vi "RMS (Half Cycle).vi"(0 "waveforms":waveform(dbl)[](array[waveform]), 1 "reset? (F)":bool, 5 "zero crossing":cluster{"zero crossing":dbl[]}[](array[cluster]), 9 "system info in":refnum<class "EP System Info.lvclass">, 11 "error in (no error)":errorcluster) -> (4 "one-cycle RMS":T1(array[cluster]), 6 "half-cycle RMS":T1(array[cluster]), 10 "system info out":refnum<class "EP System Info.lvclass">, 15 "error out":errorcluster)   [LabVIEW 2014, in "NI_EP_Power Quality.lvlib"]
doc: "Calculates the RMS voltage or RMS current for a half/single-cycle block, by using the zero crossings. You can use the Zero Crossing VI to calculate <B>zero crossing</B>. This VI refreshes the RMS values every half-cycle. You use the half/single-cycle RMS values only for detection of voltage dips, swells, and interruption events, detection of rapid voltage changes, and measurement of flickers.\n\nThis VI supports measuring single-line and multiple-line systems."
uses:
  <vilib>/addons/Electrical Power/PQ/NI_EP_Power Quality.lvlib
  <vilib>/addons/Electrical Power/PQ/Common/Classes/System Info/EP System Info.lvclass
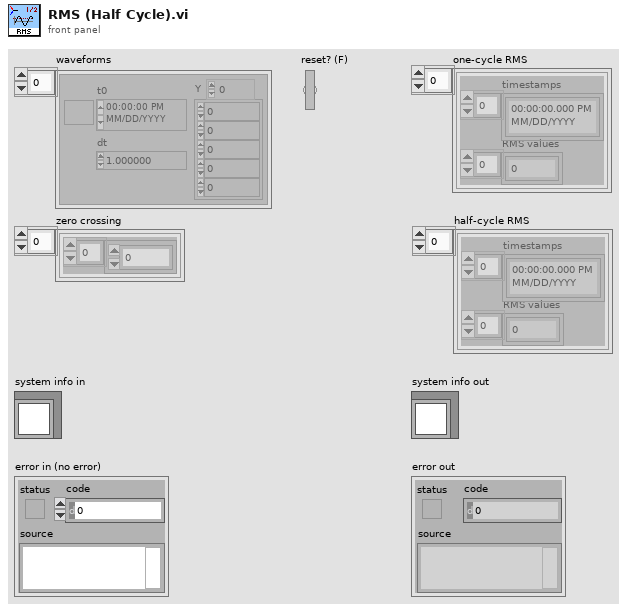
[diagram p1: front panel]
types:
  T1 = cluster{"timestamps":timestamp[], "RMS values":dbl[]}[]
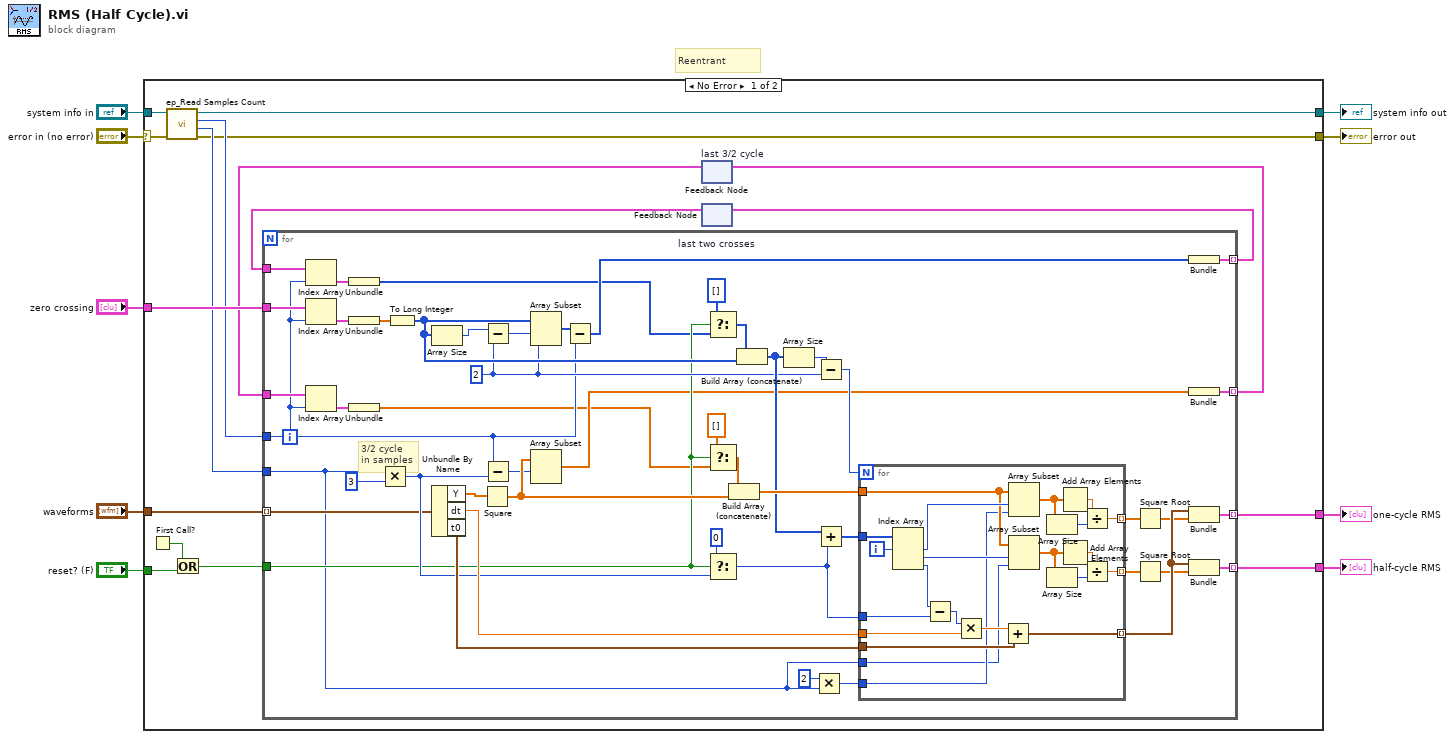
[diagram p0: block diagram]
diagram:
  # "Reentrant"
  n1 = case shown="No Error" "error in (no error)" {
    selector: "error in (no error)" -> [w19 w100]
    tunnel: "waveforms" -> [w26 _]
    tunnel: "system info in" -> [w14 w99]
    tunnel: [w20 w100] -> w5
    tunnel: [w25 _] -> w6
    tunnel: [w24 _] -> w7
    tunnel: "reset? (F)" -> [w11 _]
    tunnel: "zero crossing" -> [w23 _]
    tunnel: [w13 w99] -> w1
    frame No Error {
      n2 = First Call?() -> (First Call?: T/F=w12:bool)
      n3 = call <vilib>:"ep_Read Samples Count.vi"("error in (no error)"=w19, "system info in"=w14) -> ("error out"=w20:errorcluster, "half-cycle (samples)"=w21:i32, "basic calc. interval (samples)"=w22:i32, "system info out"=w13:refnum<class "EP System Info.lvclass">)  [unwired: 5 in, 1 out]
      n4 = Or(x=w12, y=w11) -> (x .or. y?=w10:bool)
      n5 = feedback #1 "last 3/2 cycle"() -> (w15:cluster{dbl[]}[])  [unwired: 1 in]
      n6 = feedback #2 "last two crosses"() -> (w17:cluster{i32[]}[])  [unwired: 1 in]
      n7 = for {
        tunnel: w26 -> [w46] mode=indexing
        tunnel: [w43] -> w24 mode=indexing
        tunnel: [w44] -> w25 mode=indexing
        tunnel: w10 -> [w45]
        tunnel: w23 -> [w49]
        tunnel: w22 -> [w37]
        tunnel: w21 -> [w27]
        tunnel: [w41] -> w18 mode=indexing
        tunnel: w17 -> [w39]
        tunnel: [w35] -> w16 mode=indexing
        tunnel: w15 -> [w33]
        i -> [w32]
        w56 = 2 ("length")
        # "3/2 cycle\nin samples"
        n8 = Index Array(array=w39, index=w32) -> (element=w40:cluster{i32[]})
        n9 = Index Array(array=w49, index=w32) -> (element=w48:cluster{"zero crossing":dbl[]})
        n10 = Index Array(array=w33, index=w32) -> (element=w34:cluster{dbl[]})
        n11 = Unbundle(w40) -> (w38:i32[])
        n12 = Unbundle(w48) -> ("zero crossing"=w47:dbl[])
        n13 = Unbundle(w34) -> (w31:dbl[])
        n14 = Multiply(x=w27, y=3) -> (x*y=w55:i32)
        n15 = To Long Integer(number=w47) -> (32bit integer=w58:i32[])
        n16 = Array Size(array=w58) -> (size(s)=w64:i32)
        n17 = Unbundle By Name(w46) -> ("Y"=w72:dbl[], "dt"=w71:dbl, "t0"=w70:timestamp)
        n18 = Square(x=w72) -> (x^2=w74:dbl[])
        n19 = Subtract(x=w64, y=w56) -> (x-y=w66:i32)
        n20 = Subtract(x=w37, y=w55) -> (x-y=w73:i32)
        n21 = Array Subset(array=w58, index=w66, length=w56) -> (w65:i32[])
        n22 = Array Subset(array=w74, index=w73) -> (w36:dbl[])  [unwired: 1 in]
        n23 = Subtract(x=w65, y=w37) -> (x-y=w42:i32[])
        n24 = Select(t=i32[] [], s=w45, f=w38) -> (s? t:f=w51:i32[])
        n25 = Select(t=dbl[] [], s=w45, f=w31) -> (s? t:f=w53:dbl[])
        n26 = Select(t=0 ("f"), s=w45, f=w55) -> (s? t:f=w59:i32)
        n27 = Build Array (concatenate)(w53, w74) -> (w75:dbl[])
        n28 = Build Array (concatenate)(w51, w58) -> (w61:i32[])
        n29 = Array Size(array=w61) -> (size(s)=w63:i32)
        n30 = Multiply(x=2 ("y"), y=w27) -> (x*y=w28:i32)
        n31 = Subtract(x=w63, y=w56) -> (x-y=w62:i32)
        n32 = Add(x=w61, y=w59) -> (x+y=w60:i32[])
        n33 = for {
          N: w62 -> [_]
          tunnel: w75 -> [w91]
          tunnel: w60 -> [w98]
          tunnel: [w79] -> w69 mode=indexing
          tunnel: [w80] -> w67 mode=indexing
          tunnel: w71 -> [w87]
          tunnel: w70 -> [w85]
          tunnel: [w84] -> w68 mode=indexing
          tunnel: w59 -> [w82]
          tunnel: w28 -> [w78]
          tunnel: w27 -> [w77]
          i -> [w94]
          n34 = Index Array(array=w98, index #1=w94) -> (element #1=w93:i32, element #2=w92:i32, element #3=w83:i32)  [unwired: 2 in]
          n35 = Subtract(x=w83, y=w82) -> (x-y=w81:i32)
          n36 = Multiply(x=w81, y=w87) -> (x*y=w86:dbl)
          n37 = Add(x=w86, y=w85) -> (x+y=w84:timestamp)
          n38 = Array Subset(array=w91, index=w93, length=w78) -> (w97:dbl[])
          n39 = Array Subset(array=w91, index=w92, length=w77) -> (w88:dbl[])
          n40 = Array Size(array=w97) -> (size(s)=w95:i32)
          n41 = Array Size(array=w88) -> (size(s)=w90:i32)
          n42 = Add Array Elements(numeric array=w97) -> (sum=w96:dbl)
          n43 = Add Array Elements(numeric array=w88) -> (sum=w89:dbl)
          n44 = Divide(x=w96, y=w95) -> (x/y=w79:dbl)
          n45 = Divide(x=w89, y=w90) -> (x/y=w80:dbl)
        }
        n46 = Square Root(x=w69) -> (sqrt(x)=w57:dbl[])
        n47 = Square Root(x=w67) -> (sqrt(x)=w30:dbl[])
        n48 = Bundle(w42) -> (w41:cluster{i32[]})  [unwired: 1 in]
        n49 = Bundle(w36) -> (w35:cluster{dbl[]})  [unwired: 1 in]
        n50 = Bundle(w68, w57) -> (w44:cluster{timestamp[], dbl[]})  [unwired: 1 in]
        n51 = Bundle(w68, w30) -> (w43:cluster{timestamp[], dbl[]})  [unwired: 1 in]
      }
      n52 = feedback-in #1(w16) -> ()
      n53 = feedback-in #2(w18) -> ()
    }
    frame Error {
    }
  }
  "error out" <- w5
  "one-cycle RMS" <- w6
  "system info out" <- w1
  "half-cycle RMS" <- w7
